vi "TimeSampleVI.vi"(7 "定时采样信息D":string[][](array[string]), 8 "错误输入（无错误）":errorcluster, 9 "TimeSample":refnum<user-event>, 10 "开启定时采样":bool, 11 "定时采样设置":T1 {"时" items=["1", "2", "3", "4", "5", "6", "7", "8", "9", "10", "11", "12", "13", "14", "15", "16", "17", "18", "19", "20", "21", "22", "23", "24"]; "分钟" items=["0", "1", "2", "3", "4", "5", "6", "7", "8", "9", "10", "11", "12", "13", "14", "15", "16", "17", "18", "19", "20", "21", "22", "23", "24", "25", "26", "27", "28", "29", "30", "31", "32", "33", "34", "35", "36", "37", "38", "39", "40", "41", "42", "43", "44", "45", "46", "47", "48", "49", "50", "51", "52", "53", "54", "55", "56", "57", "58", "59"]}) -> (0 "错误输出":errorcluster, 1 "hour":i32, 5 "布尔":bool)   [LabVIEW 2014, in "Sample.lvlib"]
uses:
  Sample.lvlib
panel:
  out "minute":i32
  out "second":i32
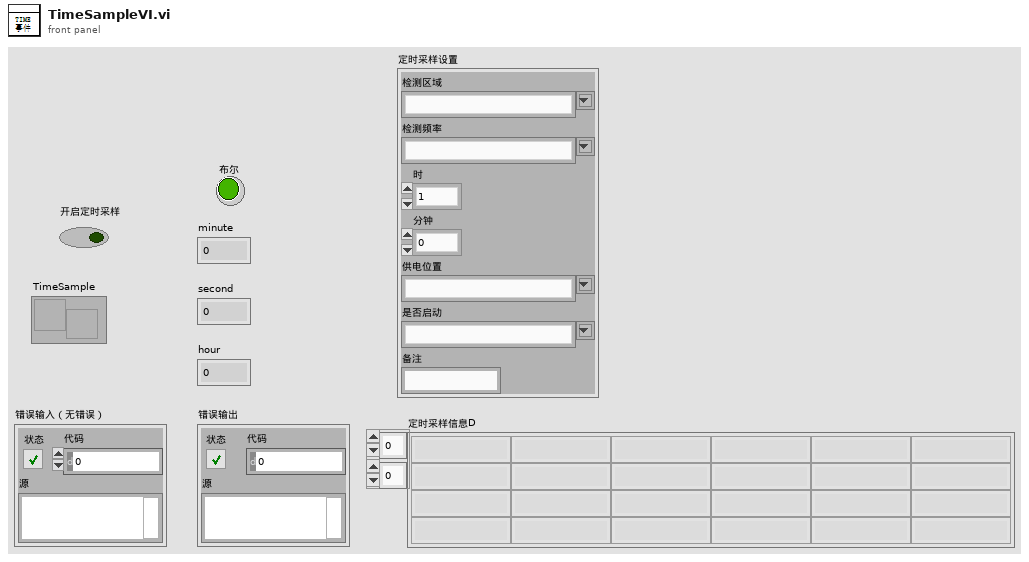
[diagram p1: front panel]
types:
  T1 = cluster{"检测区域":string, "检测频率":string, "时":u16, "分钟":u16, "供电位置":string, "是否启动":string, "备注":string}
  T2 = cluster{"区域名称":string, "采样位置":string, "采样时间":string, "时":string, "分":string}
  T3 = cluster{"分":bool, "秒":bool, "时":bool, "时 2":string, "分 2":string, "是否启动":string}
  T4 = typedef "LVDateTimeRec.ctl" = cluster{"fractional second":dbl, "second":i32, "minute":i32, "hour":i32, "day of month":i32, "month":i32, "year":i32, "day of week":i32, "day of year":i32, "DST":i32}
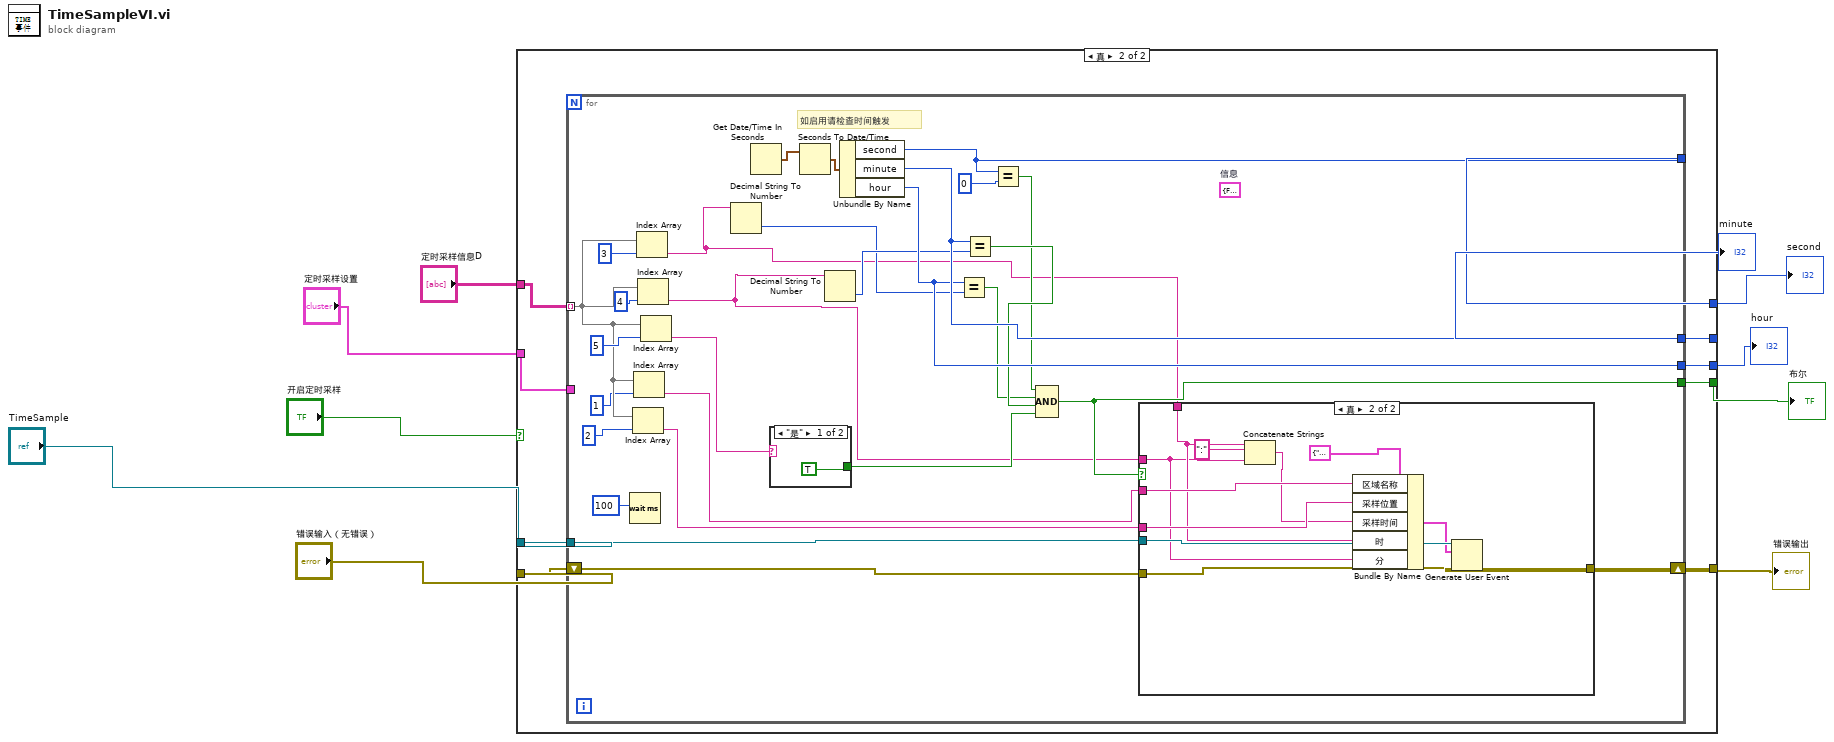
[diagram p0: block diagram]
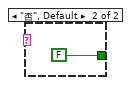
[diagram p3: hidden frame]
diagram:
  n1 = case shown="真" "开启定时采样" {
    tunnel: "TimeSample" -> [_ w20]
    tunnel: "错误输入（无错误）" -> [w11 w19]
    tunnel: [w11 w18] -> w6
    tunnel: [_ w17] -> w7
    tunnel: [_ w16] -> w8
    tunnel: [_ w15] -> w9
    tunnel: [_ w14] -> w10
    tunnel: "定时采样设置" -> [_ w12]
    tunnel: "定时采样信息D" -> [_ w13]
    frame False {
    }
    frame True {
      n2 = for {
        tunnel: w20 -> [w48]
        tunnel: [w34] -> w17
        tunnel: [w43] -> w16
        tunnel: [w41] -> w15
        tunnel: [w42] -> w14
        tunnel: w12 -> [_]
        shift-right: [w46] -> w18
        shift-left: w19 -> [w47]
        tunnel: w13 -> [w25] mode=indexing
        (unwired) T3 {"分"=FALSE, "秒"=FALSE, "时"=FALSE, "时 2"="", "分 2"="", "是否启动"=""}  # 信息
        # "如启用请检查时间触发"
        n3 = Wait (ms)(milliseconds to wait=100) -> ()  [unwired: 1 out]
        n4 = Index Array(array=w25, index=2) -> (element=w21:string)
        n5 = Index Array(array=w25, index=1) -> (element=w22:string)
        n6 = Index Array(array=w25, index=3 ("索引")) -> (element=w27:string)
        n7 = Index Array(array=w25, index=4 ("索引")) -> (element=w26:string)
        n8 = Index Array(array=w25, index=5 ("索引")) -> (element=w30:string)
        n9 = Decimal String To Number(string=w27) -> (number=w28:i32)  [unwired: 2 in, 1 out]
        n10 = Get Date/Time In Seconds() -> (seconds since 1Jan1904=w44:timestamp)
        n11 = case shown="\"是\"" w30 {
          tunnel: [TRUE FALSE] -> w38
          frame "是" {
          }
          frame "否", Default {
          }
        }
        n12 = Seconds To Date/Time(time stamp (now)=w44) -> (date time rec=w45:T4)  [unwired: 1 out]
        n13 = Decimal String To Number(string=w26) -> (number=w29:i32)  [unwired: 2 in, 1 out]
        n14 = Unbundle By Name(w45) -> ("second"=w41:i32, "minute"=w43:i32, "hour"=w42:i32)
        n15 = Equal?(x=w42, y=w28) -> (x = y?=w35:bool)
        n16 = Equal?(x=w43, y=w29) -> (x = y?=w37:bool)
        n17 = Equal?(x=w41, y=0) -> (x = y?=w36:bool)
        n18 = Compound Arithmetic op=AND(w36, w35, w37, w38) -> (w34:bool)
        n19 = case shown="真" w34 {
          tunnel: w48 -> [_ w62]
          tunnel: w47 -> [w51 w61]
          tunnel: [w51 w60] -> w46
          tunnel: w27 -> [_ w54]
          tunnel: w26 -> [_ w53]
          tunnel: w22 -> [_ w57]
          tunnel: w21 -> [_ w56]
          frame False {
          }
          frame True {
            n20 = Concatenate Strings(w54, ":", w53) -> (w55:string)
            n21 = Bundle By Name(cluster=T2 {"区域名称"="", "采样位置"="", "采样时间"="", "时"="", "分"=""} ("定时采样Info"), "区域名称"=w57, "采样位置"=w56, "采样时间"=w55, "时"=w54, "分"=w53) -> (w52:T2)
            n22 = Generate User Event(user event=w62, event data cluster=w52, error in=w61) -> (error out=w60:errorcluster)  [unwired: 1 in, 1 out]
          }
        }
      }
    }
  }
  "hour" <- w10
  "second" <- w9
  "minute" <- w8
  "布尔" <- w7
  "错误输出" <- w6
